vi "test Get Set Master RIO.vi"(8 "error in (no error)":errorcluster, 11 "TestCase in":refnum<class "Scripting API Test Case.lvclass">) -> (0 "error out":errorcluster, 3 "TestCase out":refnum<class "Scripting API Test Case.lvclass">)   [LabVIEW 2015, in "Scripting API Test Case.lvclass"]
uses:
  Scripting API Test Case.lvclass
  Scripting API/Custom Device/Engine Simulation Toolkit Custom Device Settings.ctl
  Scripting API/Bitfile/Bitfile.ctl
  NationalInstruments.VeriStand.SystemDefinitionAPI
  <userlib>/_OpenG.lib/file/file.llb/Append Path to Root if Relative - Scalar__ogtk.vi
  <vilib>/addons/_JKI Toolkits/VI Tester/TestCase.llb/TestCase.lvclass
  niveristand-custom-device-testing-tools/VeriStandTestUtilities/VeriStandTestUtilities.lvlib
  Scripting API/Engine Simulation Toolkit Scripting API.lvlib
panel:
  in  "Save?":bool
  out "Output Filename":string
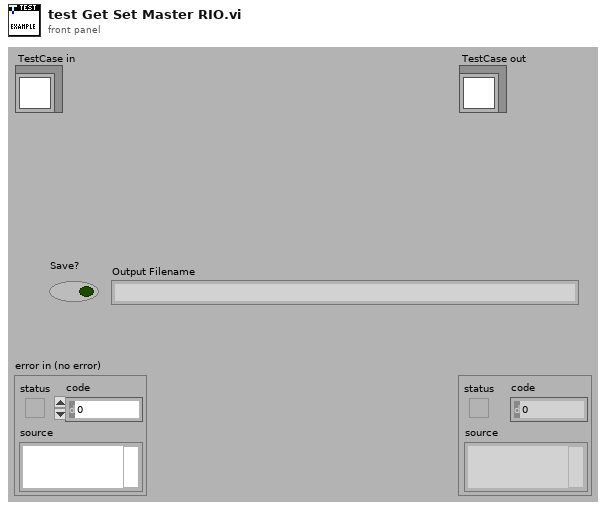
[diagram p1: front panel]
types:
  T1 = typedef "Engine Simulation Toolkit Scripting API.lvlib/Bitfile.ctl" = cluster{"RIO Device Address":string, "Bitfile Path":path}
  T2 = typedef "Engine Simulation Toolkit Scripting API.lvlib/Engine Simulation Toolkit Custom Device Settings.ctl" = cluster{"Name":string, "Execution priority":enum16{"Low", "Medium", "High"}, "Rate decimation":i32, "CPU":i32}
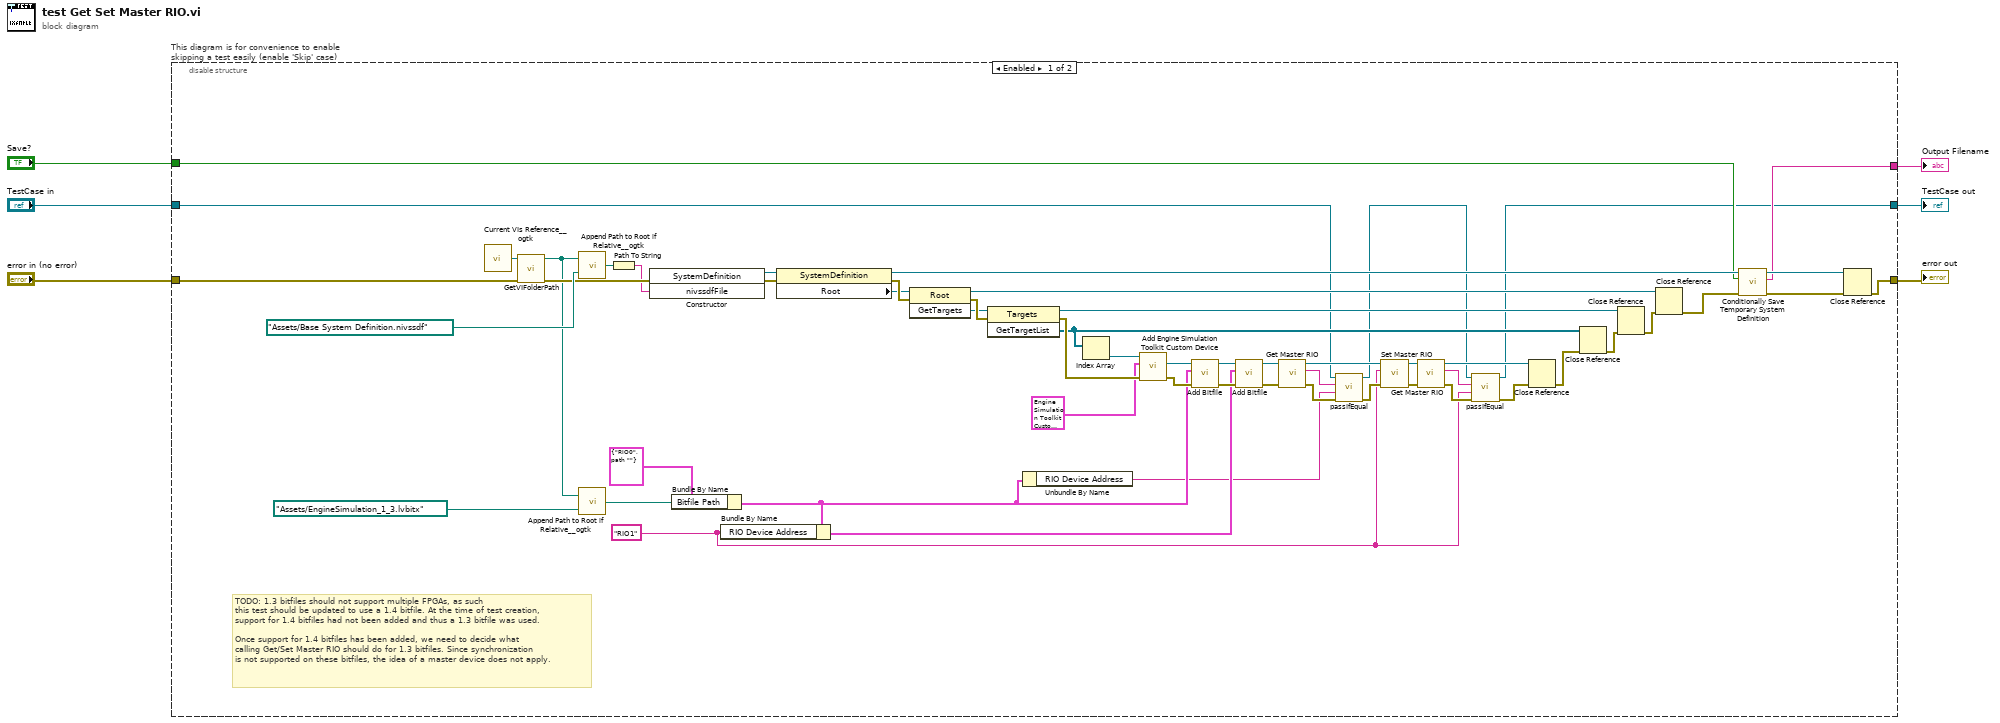
[diagram p0: block diagram]
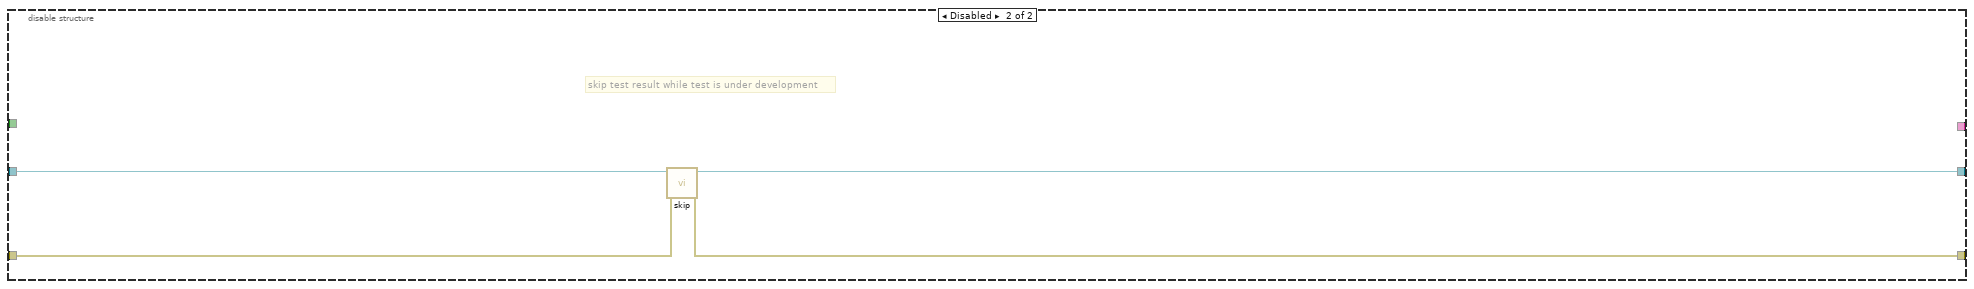
[diagram p2: hidden frame]
diagram:
  n1 = disable-structure "This diagram is for convenience to enable skipping a test easily (enable 'Skip' case)" shown="Enabled" {
    disable-tunnel: "TestCase in" -> [w8 w65]
    disable-tunnel: [w9 w63] -> w3
    disable-tunnel: [w53 w64] -> w5
    disable-tunnel: "error in (no error)" -> [w60 w62]
    disable-tunnel: [w36 _] -> w2
    disable-tunnel: "Save?" -> [w35 _]
    frame Enabled {
      w11 = "RIO1" ("RIO Device Address")
      # "TODO: 1.3 bitfiles should not support multiple FPGAs, as such\nthis test should be updated to use a 1.4 bitfile. At the time of test creation,\nsupport for 1.4 bitfiles had not been added and thus a 1.3 bitfile was used.\n\nOnce support for 1.4 bitfiles has been added, we need to decide what\ncalling Get/Set Master RIO should do for 1.3 bitfiles. Since synchronization\nis not supported on these bitfiles, the idea of a master device does not apply."
      n2 = call <userlib>:"Current VIs Reference__ogtk.vi"() -> ("Current VI's reference"=w61:refnum<vi>)  [unwired: 5 in]
      n3 = call "GetVIFolderPath.vi"("error in (no error)"=w60, "VI Reference in"=w61) -> ("error out"=w57:errorcluster, "VI Folder Path out"=w31:path)  [unwired: 8 in]
      n4 = call-poly <userlib>:"Append Path to Root if Relative__ogtk.vi"("Absolute or Relative Path"=path "Assets/Base System Definition.nivssdf", "Root Path"=w31) -> ("Absolute or Appended Path"=w58:path)
      n5 = call-poly <userlib>:"Append Path to Root if Relative__ogtk.vi"("Absolute or Relative Path"=path "Assets/EngineSimulation_1_3.lvbitx", "Root Path"=w31) -> ("Absolute or Appended Path"=w28:path)
      n6 = Path To String(path=w58) -> (string=w55:string)
      n7 = constructor class="SystemDefinition"(error in=w57, "nivssdfFile"=w55) -> (reference out=w54:refnum<k24>, error out=w56:errorcluster)  [unwired: 2 in, 2 out]
      n8 = Bundle By Name(cluster=T1 {"RIO Device Address"="RIO0", "Bitfile Path"=path ""} ("Engine Simulation Toolkit Bitfile"), "Bitfile Path"=w28) -> (w20:T1)
      n9 = Bundle By Name(cluster=w20, "RIO Device Address"=w11) -> (w26:T1)
      n10 = property class="SystemDefinition"(reference=w54, error in=w56) -> (reference out=w38:refnum<k24>, error out=w51:errorcluster, "Root"=w50:refnum<k24>)
      n11 = invoke class="Root" method="GetTargets"(reference=w50, error in=w51) -> (reference out=w52:refnum<k24>, error out=w47:errorcluster, "GetTargets"=w46:refnum<k24>)  [unwired: 1 in]
      n12 = invoke class="Targets" method="GetTargetList"(reference=w46, error in=w47) -> (reference out=w48:refnum<k24>, error out=w43:errorcluster, "GetTargetList"=w42:refnum<k24>[])  [unwired: 1 in]
      n13 = Unbundle By Name(w20) -> ("RIO Device Address"=w19:string)
      n14 = Index Array(array=w42) -> (element=w44:refnum<k24>)  [unwired: 1 in]
      n15 = call "Add Engine Simulation Toolkit Custom Device.vi"("error in (no error)"=w43, "Settings"=T2 {"Name"="Engine Simulation Toolkit Custom Device", "Execution priority"=enum."Medium", "Rate decimation"=1, "CPU"=-2} ("Engine Simulation Toolkit Custom Device Settings"), "Target in"=w44) -> ("error out"=w32:errorcluster, "EST Custom Device"=w34:refnum<k24>)  [unwired: 6 in, 1 out]
      n16 = call "Add Bitfile.vi"("error in (no error)"=w32, "Engine Simulation Toolkit Bitfile"=w20, "EST Custom Device in"=w34) -> ("error out"=w27:errorcluster, "EST Custom Device out"=w25:refnum<k24>)  [unwired: 7 in]
      n17 = call "Add Bitfile.vi"("error in (no error)"=w27, "Engine Simulation Toolkit Bitfile"=w26, "EST Custom Device in"=w25) -> ("error out"=w24:errorcluster, "EST Custom Device out"=w23:refnum<k24>)  [unwired: 7 in]
      n18 = call "Get Master RIO.vi"("error in (no error)"=w24, "EST Custom Device in"=w23) -> ("error out"=w22:errorcluster, "RIO Device Address"=w21:string, "EST Custom Device out"=w15:refnum<k24>)  [unwired: 7 in]
      n19 = call-dynamic "passIfEqual.vi"("error in (no error)"=w22, "y"=w19, "x"=w21, "TestCase in"=w8) -> ("error out"=w18:errorcluster, "TestCase out"=w7:refnum<class "Scripting API Test Case.lvclass">)  [unwired: 6 in]
      n20 = call "Set Master RIO.vi"("error in (no error)"=w18, "RIO Device Address"=w11, "EST Custom Device in"=w15) -> ("error out"=w17:errorcluster, "EST Custom Device out"=w16:refnum<k24>)  [unwired: 7 in]
      n21 = call "Get Master RIO.vi"("error in (no error)"=w17, "EST Custom Device in"=w16) -> ("error out"=w14:errorcluster, "RIO Device Address"=w12:string, "EST Custom Device out"=w10:refnum<k24>)  [unwired: 7 in]
      n22 = call-dynamic "passIfEqual.vi"("error in (no error)"=w14, "y"=w11, "x"=w12, "TestCase in"=w7) -> ("error out"=w13:errorcluster, "TestCase out"=w9:refnum<class "Scripting API Test Case.lvclass">)  [unwired: 6 in]
      n23 = Close Reference(reference=w10, error in (no error)=w13) -> (error out=w41:errorcluster)
      n24 = Close Reference(reference=w42, error in (no error)=w41) -> (error out=w45:errorcluster)
      n25 = Close Reference(reference=w48, error in (no error)=w45) -> (error out=w49:errorcluster)
      n26 = Close Reference(reference=w52, error in (no error)=w49) -> (error out=w37:errorcluster)
      n27 = call "Conditionally Save Temporary System Definition.vi"("error in (no error)"=w37, "Save?"=w35, ".NET Refnum in"=w38) -> ("error out"=w40:errorcluster, "filename"=w36:string, ".NET Refnum out"=w39:refnum<k24>)  [unwired: 6 in]
      n28 = Close Reference(reference=w39, error in (no error)=w40) -> (error out=w53:errorcluster)
    }
    frame Disabled {
      # "skip test result while test is under development"
      n29 = call <vilib>:"skip.vi"("error in (no error)"=w62, "TestCase in"=w65) -> ("error out"=w64:errorcluster, "TestCase out"=w63:refnum<class "Scripting API Test Case.lvclass">)  [unwired: 8 in]
    }
  }
  "error out" <- w5
  "TestCase out" <- w3
  "Output Filename" <- w2
